vi "CreateSeriesMapFile.vi"() -> ()   [LabVIEW 2024]
panel:
  in  "Filter":string
  out "Current State":string
  in  "save key set":bool
  in  "match selected":bool
  in  "Marvel Series":i32(listbox)
  in  "Marvel Filter":i32(listbox)
  in  "CLZ Series":i32(listbox)
  in  "CLZ Filter":i32(listbox)
  in  "Exit":bool
  # "#TODO: Add Hunters fuzzy toolkit"
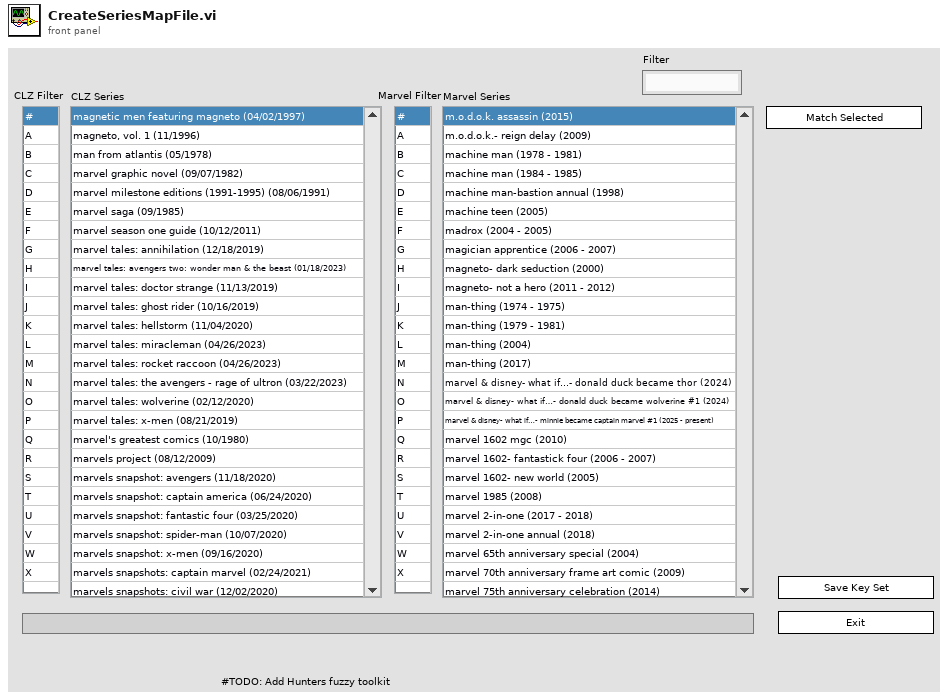
[diagram p1: front panel]
types:
  T1 = enum32{"Invalid", "Standard", "Closed", "Hidden", "Minimized", "Maximized"}
  T2 = enum32{"invalid app kind", "Development System", "Run Time System", "Student Edition", "Embedded LabVIEW", "Evaluation", "Custom"}
  T3 = cluster{"Core":cluster{"Current VI Reference":refnum<vi>, "Close Panel on Exit?":bool}, "marvel series map":map{i32, string}, "clz series map":map{i32, cluster{"series title":string, "pub date":string}}, "filtered clz map":map{string, i32}, "filtered marvel map":map{string, i32}, "key set":set{cluster{"clz.key":i32, "marvel.key":i32}}}
  T4 = map{i32, cluster{"series title":string, "pub date":string}}
  T5 = cluster{"Current VI Reference":refnum<vi>, "Close Panel on Exit?":bool}
  T6 = cluster{"key_pairs":cluster{"clz.key":i32, "marvel.key":i32}[]}
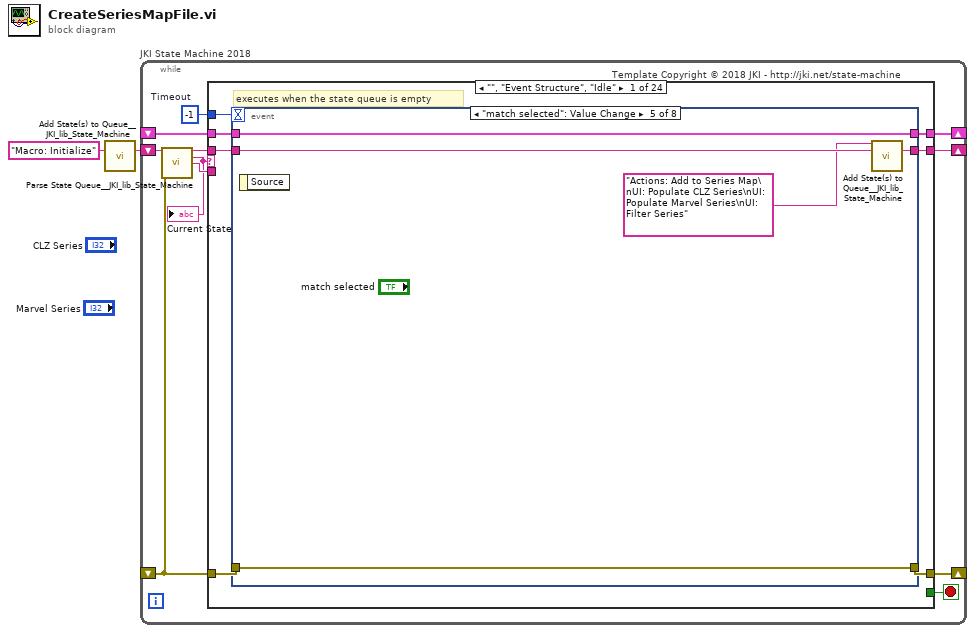
[diagram p0: block diagram]
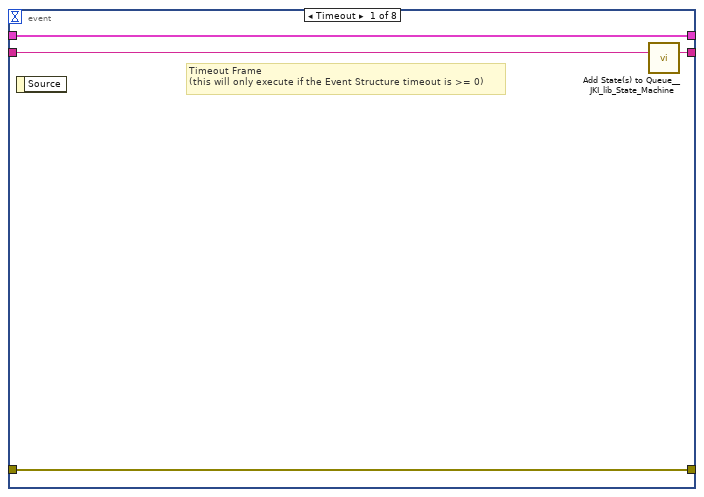
[diagram p2: hidden frame]
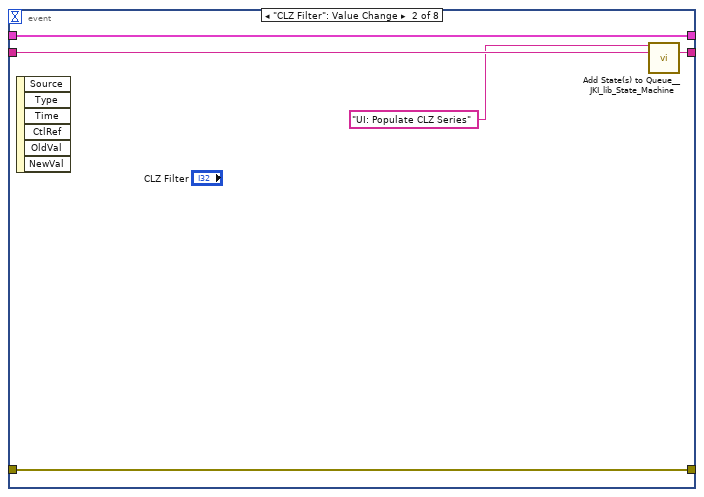
[diagram p3: hidden frame]
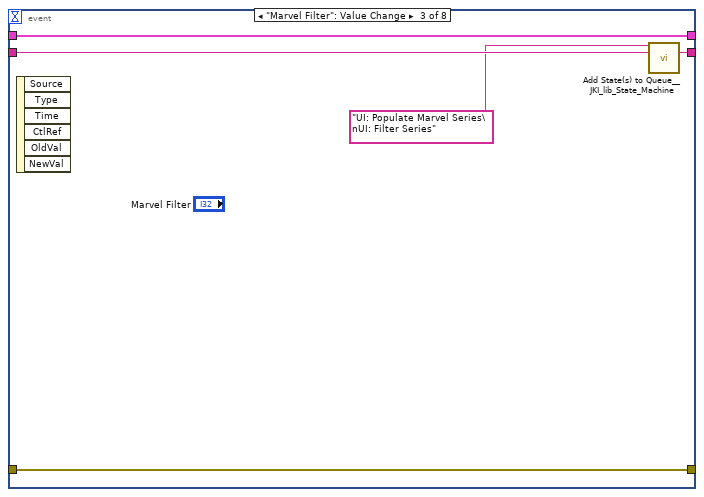
[diagram p4: hidden frame]
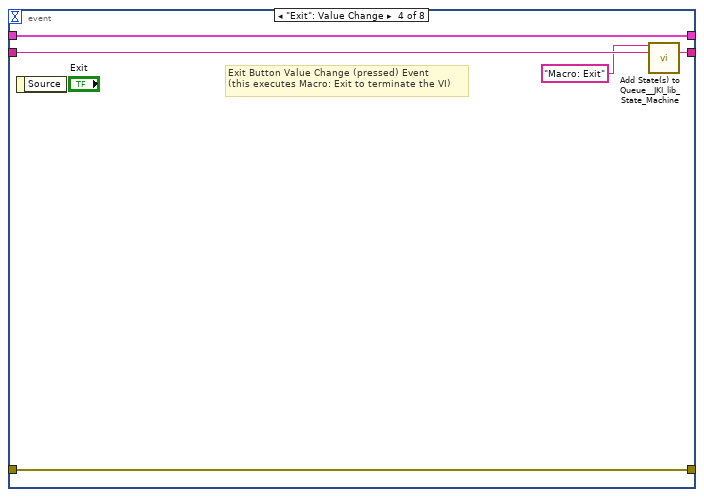
[diagram p5: hidden frame]
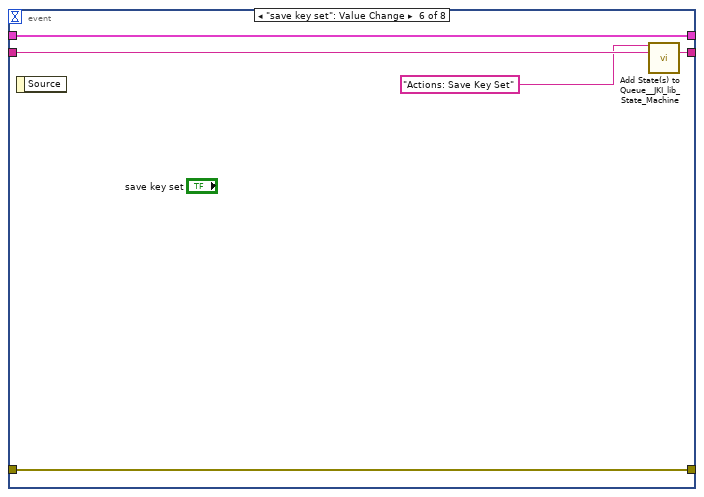
[diagram p6: hidden frame]
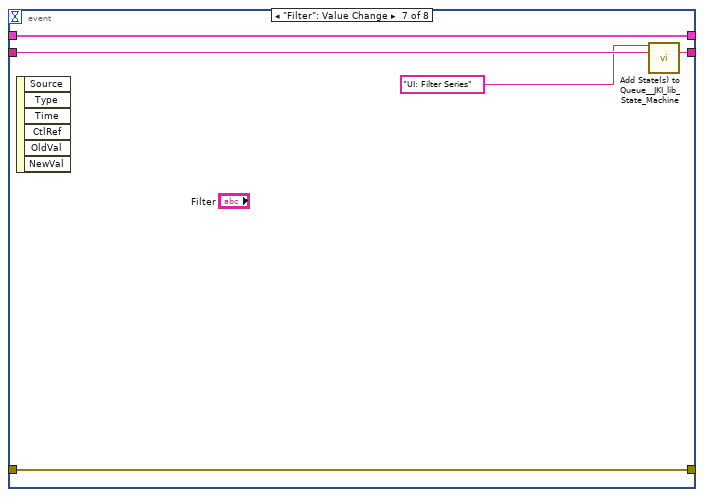
[diagram p7: hidden frame]
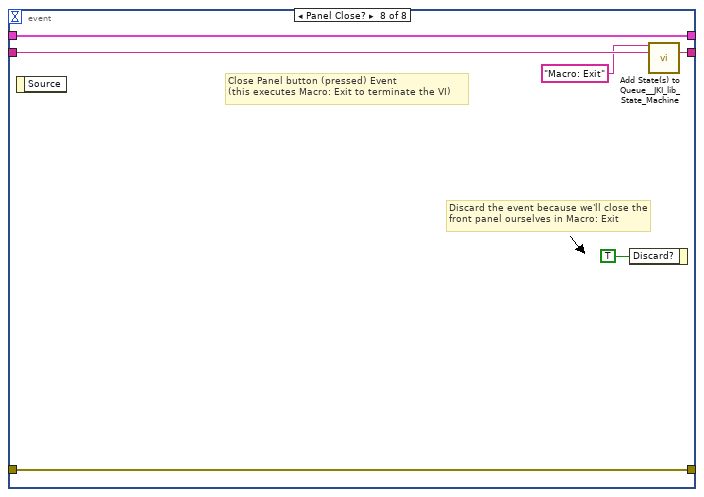
[diagram p8: hidden frame]
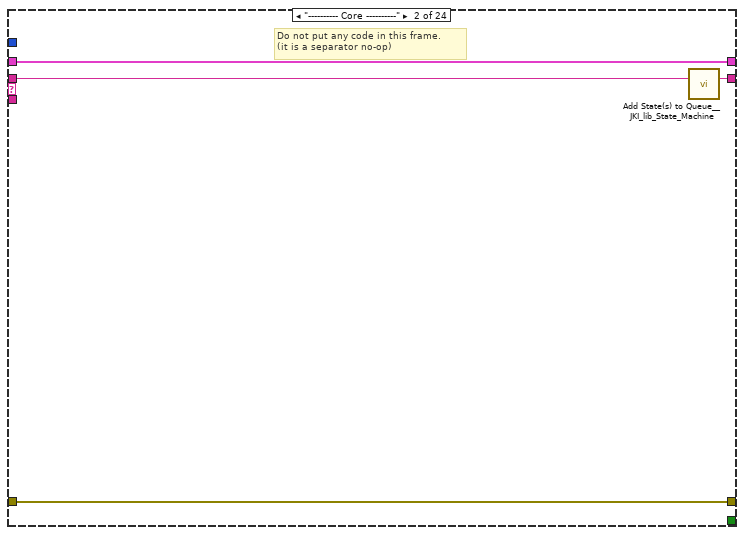
[diagram p9: hidden frame]
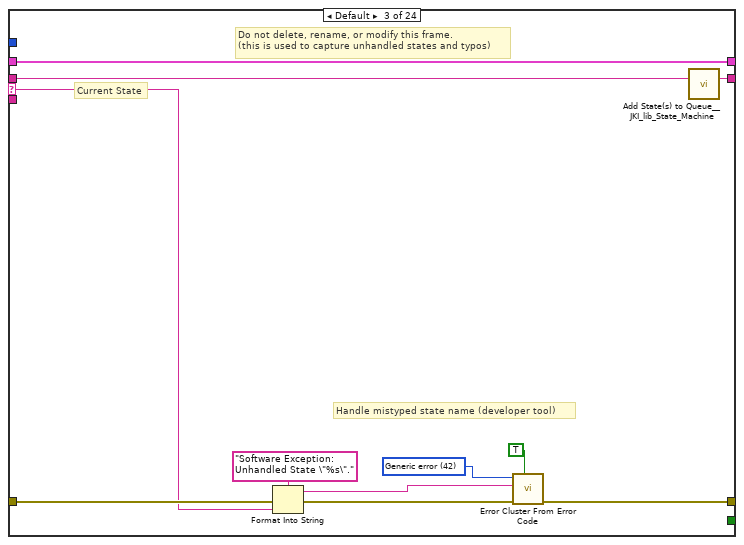
[diagram p10: hidden frame]
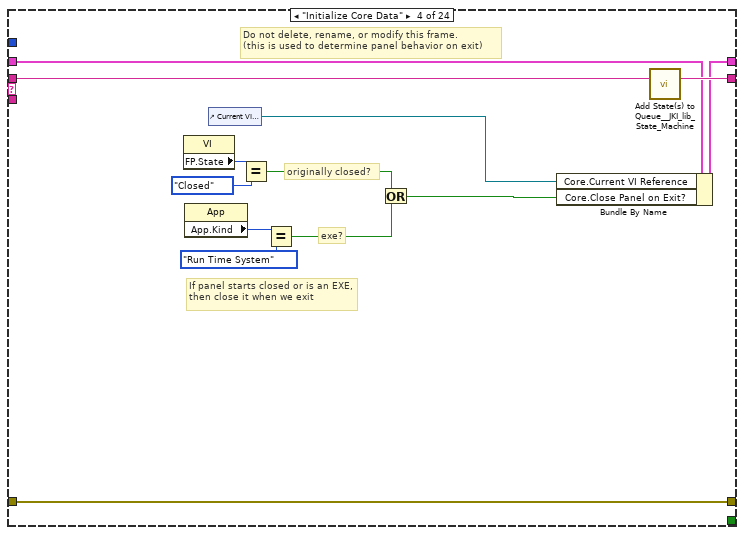
[diagram p11: hidden frame]
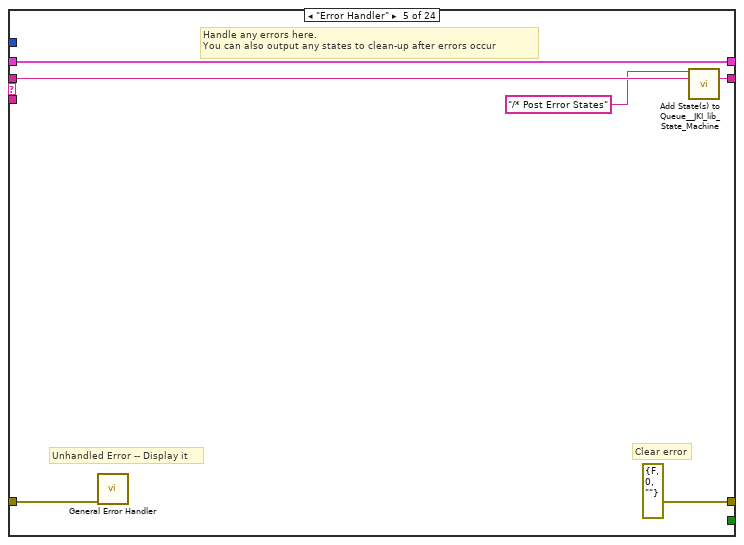
[diagram p12: hidden frame]
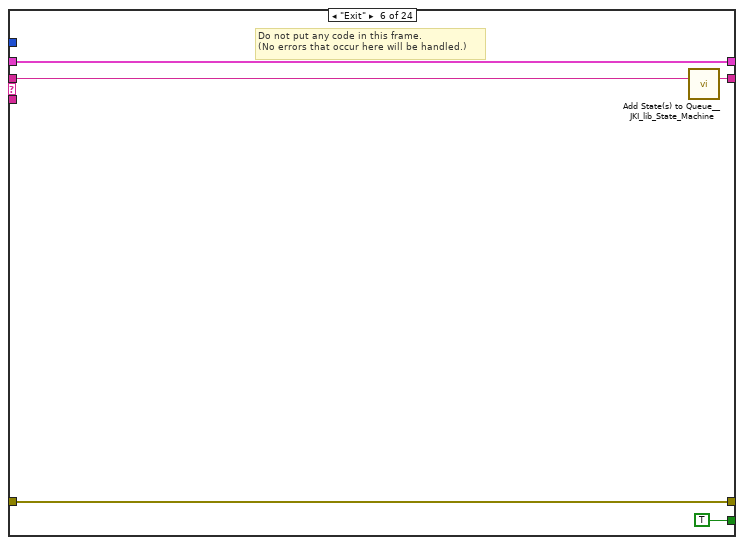
[diagram p13: hidden frame]
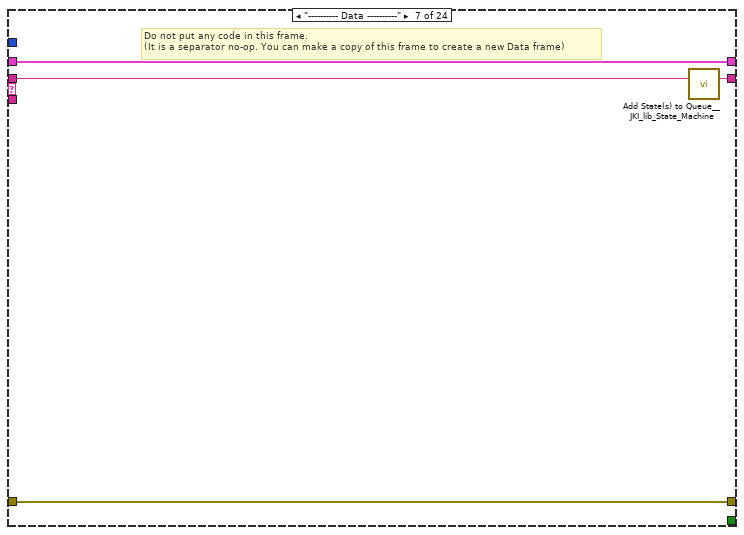
[diagram p14: hidden frame]
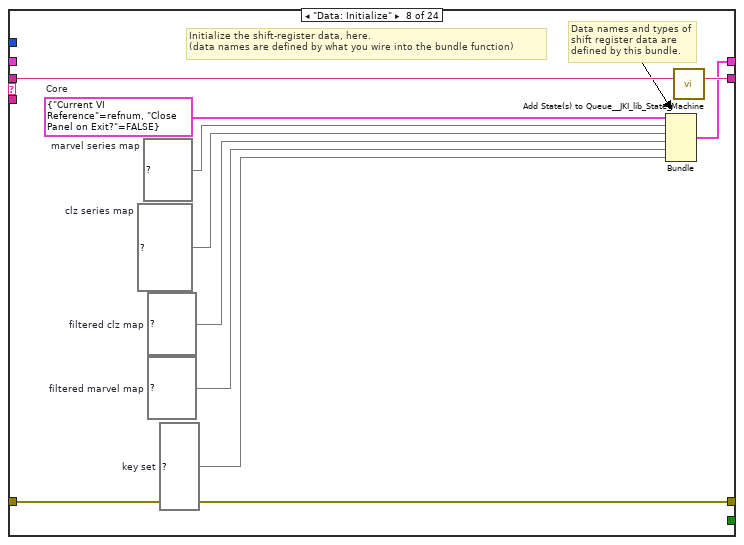
[diagram p15: hidden frame]
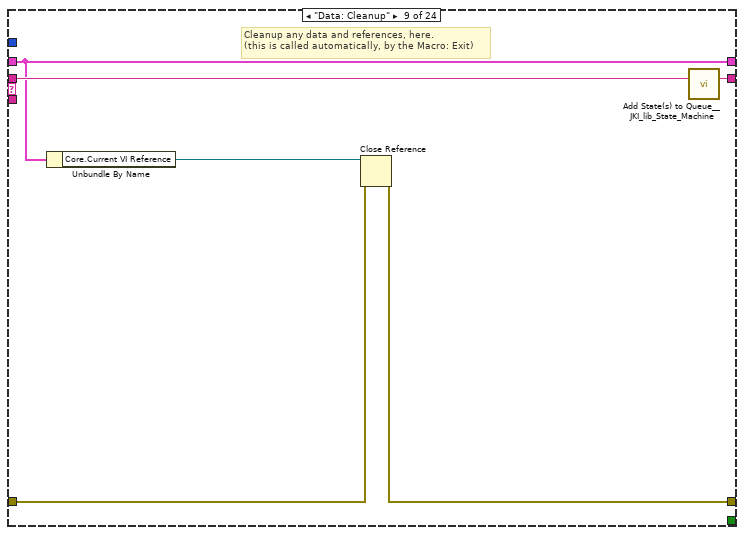
[diagram p16: hidden frame]
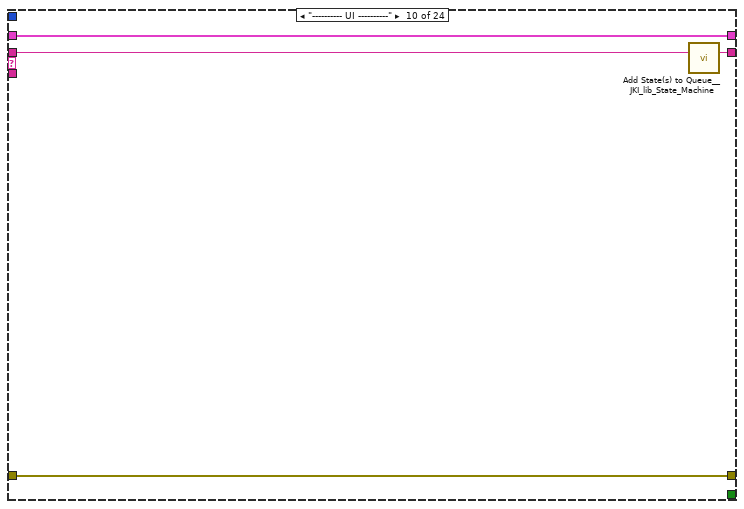
[diagram p17: hidden frame]
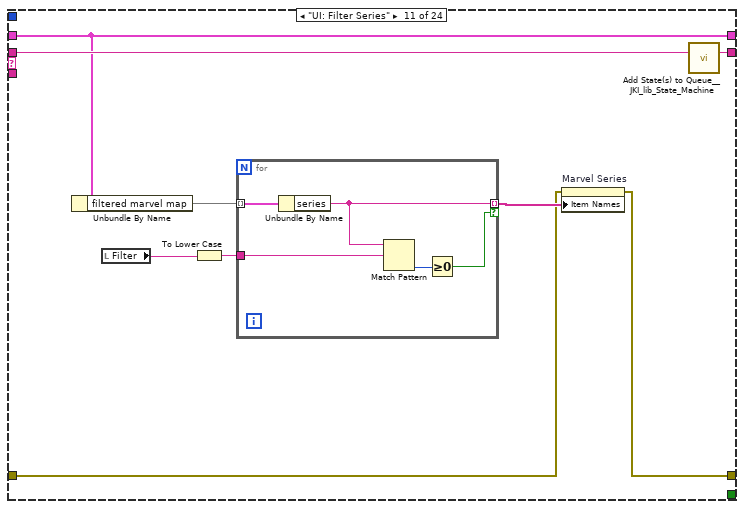
[diagram p18: hidden frame]
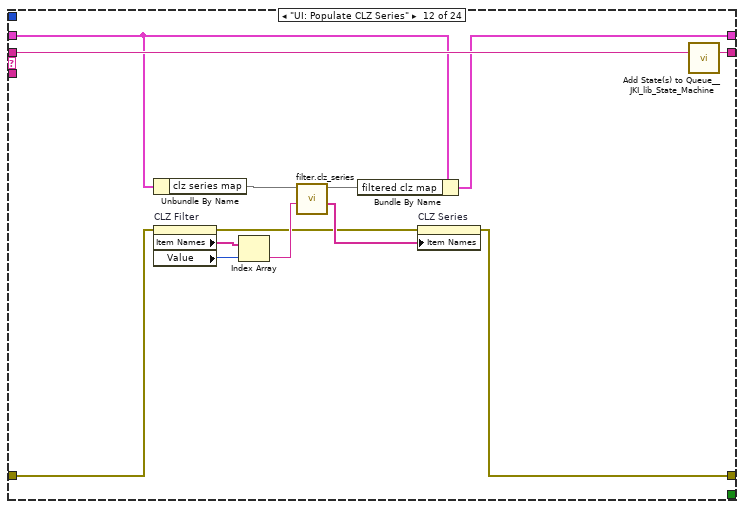
[diagram p19: hidden frame]
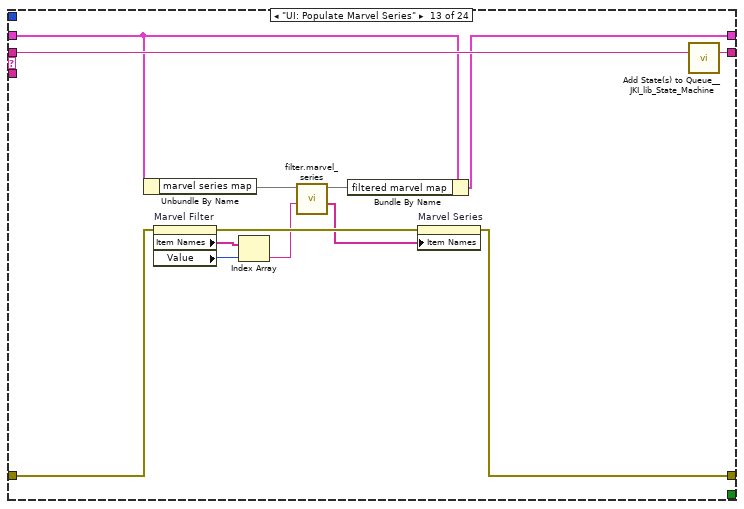
[diagram p20: hidden frame]
diagram:
  n1 = call <vilib>:"Add State(s) to Queue__JKI_lib_State_Machine.vi"("State(s) in (\"\")"="Macro: Initialize") -> ("States Out"=w2:string)  [unwired: 14 in]
  n2 = while "JKI State Machine 2018" {
    shift-right: [w7] -> _
    shift-left: _ -> [w6]
    shift-right: [w10] -> _
    shift-left: _ -> [w4]
    shift-right: [w9] -> _
    shift-left: w2 -> [w11]
    stop <- w8 stop-if-true
    w5 = -1  # Timeout
    # "Template Copyright © 2018 JKI - http://jki.net/state-machine"
    n3 = call <vilib>:"Parse State Queue__JKI_lib_State_Machine.vi"("State Queue"=w11, "Error In (no error)"=w4) -> ("Remaining States"=w13:string, "Current State"=w3:string, "Arguments"=w12:string)  [unwired: 11 in]
    "Current State" <- w3
    n4 = case shown="\"\", \"Event Structure\", \"Idle\"" w3 {
      selector: w3 -> [_ _ w65 _ _ _ _ _ _ _ _ _ _ _ _ _ _ _ _ _ _ _ _ _]
      tunnel: w13 -> [w20 w64 w69 w88 w94 w99 w103 w113 w119 w123 w132 w150 w163 w173 w179 w190 w259 w264 w274 w278 w289 w300 w316 w336]
      tunnel: w12 -> [_ _ _ _ _ _ _ _ _ _ _ _ _ _ w174 w184 _ _ _ _ _ _ _ _]
      tunnel: w6 -> [w18 w61 w67 w81 w91 w97 w100 _ w114 w120 w128 w140 w156 w171 w177 w186 w256 w261 w271 w275 w287 w292 w314 w324]
      tunnel: [w17 w62 w71 w85 errorcluster {"status"=FALSE, "code"=0, "source"=""} ("error out") w96 w101 w110 w115 w121 w124 w142 w158 w164 w175 w187 w257 w262 w272 w276 w284 w296 w301 w334] -> w10
      tunnel: w4 -> [w16 w62 w70 w85 w90 w96 w101 w110 w116 w121 w125 w141 w157 w167 w176 w188 w257 w262 w272 w276 w283 w298 w302 w334]
      tunnel: [w19 w63 w68 w87 w93 w98 w102 w112 w118 w122 w131 w149 w162 w172 w178 w189 w258 w263 w273 w277 w288 w299 w315 w335] -> w9
      tunnel: [_ _ _ _ _ TRUE _ _ _ _ _ _ _ _ _ _ _ _ _ _ _ _ _ _] -> w8
      tunnel: [w15 w61 w67 w86 w91 w97 w100 w111 w114 w120 w128 w139 w155 w171 w177 w186 w256 w261 w271 w275 w287 w295 w313 w323] -> w7
      tunnel: w5 -> [w14 _ _ _ _ _ _ _ _ _ _ _ _ _ _ _ _ _ _ _ _ _ _ _]
      frame "", "Event Structure", "Idle" {
        # "executes when the state queue is empty"
        n5 = event shown="[4] \"match selected\": Value Change" {
          selector: _ -> [_ _ _ _ _ _ _ _]
          dyn-events: _ -> [_ _ _ _ _ _ _ _]
          timeout: w14 -> [_ _ _ _ _ _ _ _]
          tunnel: w20 -> [w24 w29 w34 w39 w44 w49 w54 w60]
          tunnel: [w23 w28 w33 w38 w43 w48 w53 w59] -> w19
          tunnel: w18 -> [w21 w26 w31 w36 w41 w46 w51 w57]
          tunnel: [w22 w27 w32 w37 w42 w47 w52 w58] -> w17
          tunnel: w16 -> [w22 w27 w32 w37 w42 w47 w52 w58]
          tunnel: [w21 w26 w31 w36 w41 w46 w51 w57] -> w15
          event Timeout {
            # "Timeout Frame\n(this will only execute if the Event Structure timeout is >= 0)"
            n6 = event-data() -> ()  [unwired: 1 in, 1 out]
            n7 = call <vilib>:"Add State(s) to Queue__JKI_lib_State_Machine.vi"("State(s) in (\"\")"=w24) -> ("States Out"=w23:string)  [unwired: 14 in]
          }
          event "CLZ Filter": Value Change {
            n8 = event-data() -> ()  [unwired: 1 in, 6 out]
            n9 = call <vilib>:"Add State(s) to Queue__JKI_lib_State_Machine.vi"("State(s) in Front (\"\")"="UI: Populate CLZ Series", "State(s) in (\"\")"=w29) -> ("States Out"=w28:string)  [unwired: 13 in]
          }
          event "Marvel Filter": Value Change {
            n10 = event-data() -> ()  [unwired: 1 in, 6 out]
            n11 = call <vilib>:"Add State(s) to Queue__JKI_lib_State_Machine.vi"("State(s) in Front (\"\")"="UI: Populate Marvel Series\nUI: Filter Series", "State(s) in (\"\")"=w34) -> ("States Out"=w33:string)  [unwired: 13 in]
          }
          event "Exit": Value Change {
            # "Exit Button Value Change (pressed) Event\n(this executes Macro: Exit to terminate the VI)"
            n12 = event-data() -> ()  [unwired: 1 in, 1 out]
            n13 = call <vilib>:"Add State(s) to Queue__JKI_lib_State_Machine.vi"("State(s) in Front (\"\")"="Macro: Exit", "State(s) in (\"\")"=w39) -> ("States Out"=w38:string)  [unwired: 13 in]
          }
          event "match selected": Value Change {
            n14 = event-data() -> ()  [unwired: 1 in, 1 out]
            n15 = call <vilib>:"Add State(s) to Queue__JKI_lib_State_Machine.vi"("State(s) in Front (\"\")"="Actions: Add to Series Map\nUI: Populate CLZ Series\nUI: Populate Marvel Series\nUI: Filter Series", "State(s) in (\"\")"=w44) -> ("States Out"=w43:string)  [unwired: 13 in]
          }
          event "save key set": Value Change {
            n16 = event-data() -> ()  [unwired: 1 in, 1 out]
            n17 = call <vilib>:"Add State(s) to Queue__JKI_lib_State_Machine.vi"("State(s) in Front (\"\")"="Actions: Save Key Set", "State(s) in (\"\")"=w49) -> ("States Out"=w48:string)  [unwired: 13 in]
          }
          event "Filter": Value Change {
            n18 = event-data() -> ()  [unwired: 1 in, 6 out]
            n19 = call <vilib>:"Add State(s) to Queue__JKI_lib_State_Machine.vi"("State(s) in Front (\"\")"="UI: Filter Series", "State(s) in (\"\")"=w54) -> ("States Out"=w53:string)  [unwired: 13 in]
          }
          event Panel Close? {
            # "Discard the event because we'll close the front panel ourselves in Macro: Exit"
            # "Close Panel button (pressed) Event\n(this executes Macro: Exit to terminate the VI)"
            n20 = event-data() -> ()  [unwired: 1 in, 1 out]
            n21 = event-data("Discard?"=TRUE) -> ()  [unwired: 1 in, 1 out]
            n22 = call <vilib>:"Add State(s) to Queue__JKI_lib_State_Machine.vi"("State(s) in Front (\"\")"="Macro: Exit", "State(s) in (\"\")"=w60) -> ("States Out"=w59:string)  [unwired: 13 in]
          }
        }
      }
      frame "---------- Core ----------" {
        # "Do not put any code in this frame.\n(it is a separator no-op)"
        n23 = call <vilib>:"Add State(s) to Queue__JKI_lib_State_Machine.vi"("State(s) in (\"\")"=w64) -> ("States Out"=w63:string)  [unwired: 14 in]
      }
      frame Default {
        w74 = 42 items=["No error", "Argument error", "Memory is full", "Out of zone", "End of file", "File already open", "Generic file I/O error", "File not found", "File permission error", "Disk is full", "Duplicate path", "Too many files open", "System feature not enabled", "Resource file not found", "Cannot add resource", "Resource not found", "Image not found", "Image memory error", "Pen does not exist", "Config type invalid", "Config token not found", "Config parse error", "Config memory error", "Bad external code format", "Bad external code offset", "External code not present", "Null window", "Destroy window error", "Null menu", "Print aborted", "Bad print record", "Print driver error", "Windows error during printing", "Memory error during printing", "Print dialog error", "Generic print error", "Invalid device refnum", "Device not found", "Device parameter error", "Device unit error", "Cannot open device", "Device call aborted", "Generic error", "Cancelled by user", "Object ID too low", "Object ID too high", "Object not in heap", "Unknown heap", "Unknown object (invalid DefProc)", "Unknown object (DefProc not in table)", "Message out of range", "Invalid (null) method", "Unknown message", "Manager call not supported", "Bad address", "Network operation in progress", "Network operation timed out", "Connection is busy", "Network attribute not supported", "Network error", "Address in use", "System out of memory", "Connection aborted", "Connection refused", "Not connected", "Already connected", "Connection closed", "Initialization error (interapplication manager)", "Bad occurrence", "Wait on unbound occurrence handler", "Occurrence queue overflow", "Datalog type conflict", "Unused", "Unrecognized type (interapplication manager)", "Memory corrupt", "Failed to make temporary DLL", "Old CIN version", "Drag socket not found", "Failed to load drop-object", "Failed to register OLE object", "Failed to release OLE object", "Format specifier type mismatch", "Unknown format specifier", "Too few format specifiers", "Too many format specifiers", "Scan failed", "Newer CIN version", "Error converting to variant", "Runtime menu error", "Password tampered", "Variant attribute not found", "Incompatible variant data type", "Event data is not available", "Event Store is not present", "Occurrence is not found", "Event Queue is not created", "Event info is not available", "Refnum passed is NULL", "Error retrieving Class GUID", "Error retrieving CoClass GUID", "Error retrieving TypeLib GUID.", "Bad built application magic bytes.", "Specific driver is different from the specific driver associated with the Logical Name.", "There is no session opened to the class driver.", "Max Error", "MAX - Error with config objects", "MAX - Error loading configuration", "MAX - Group not supported"]
        # "Current State"
        # "Do not delete, rename, or modify this frame.\n(this is used to capture unhandled states and typos)"
        # "Handle mistyped state name (developer tool)"
        n24 = Format Into String(format string="Software Exception: Unhandled State \"%s\"." ("message"), error in=w70, w65) -> (resulting string=w73:string, error out=w72:errorcluster)  [unwired: 1 in]
        n25 = call <vilib>:"Error Cluster From Error Code.vi"("show call chain? (False)"=TRUE, "error in (no error)"=w72, "error message (\"\")"=w73, "error code (0)"=w74) -> ("error out"=w71:errorcluster)  [unwired: 5 in]
        n26 = call <vilib>:"Add State(s) to Queue__JKI_lib_State_Machine.vi"("State(s) in (\"\")"=w69) -> ("States Out"=w68:string)  [unwired: 14 in]
      }
      frame "Initialize Core Data" {
        # "Do not delete, rename, or modify this frame.\n(this is used to determine panel behavior on exit)"
        # "originally closed?"
        # "exe?"
        # "If panel starts closed or is an EXE, then close it when we exit"
        n27 = property class="VI"() -> ("FP.State"=w78:T1)  [unwired: 2 in, 2 out]
        n28 = property class="App"() -> ("App.Kind"=w84:T2)  [unwired: 2 in, 2 out]
        n29 = control-ref of="Current VI Reference"() -> (w79:refnum<vi>)
        n30 = Equal?(x=w78, y=T1."Closed" ("Front Panel Window:State")) -> (x = y?=w76:bool)
        n31 = Equal?(x=w84, y=T2."Run Time System" ("Application:Kind")) -> (x = y?=w82:bool)
        n32 = Or(x=w76, y=w82) -> (x .or. y?=w80:bool)
        n33 = Bundle By Name(cluster=w81, "Core.Current VI Reference"=w79, "Core.Close Panel on Exit?"=w80) -> (w86:T3)
        n34 = call <vilib>:"Add State(s) to Queue__JKI_lib_State_Machine.vi"("State(s) in (\"\")"=w88) -> ("States Out"=w87:string)  [unwired: 14 in]
      }
      frame "Error Handler" {
        # "Unhandled Error -- Display it"
        # "Handle any errors here.\nYou can also output any states to clean-up after errors occur"
        # "Clear error"
        n35 = call <vilib>:"General Error Handler.vi"("error in (no error)"=w90) -> ()  [unwired: 10 in, 5 out]
        n36 = call <vilib>:"Add State(s) to Queue__JKI_lib_State_Machine.vi"("State(s) in Front (\"\")"="/* Post Error States", "State(s) in (\"\")"=w94) -> ("States Out"=w93:string)  [unwired: 13 in]
      }
      frame "Exit" {
        # "Do not put any code in this frame.\n(No errors that occur here will be handled.)"
        n37 = call <vilib>:"Add State(s) to Queue__JKI_lib_State_Machine.vi"("State(s) in (\"\")"=w99) -> ("States Out"=w98:string)  [unwired: 14 in]
      }
      frame "---------- Data ----------" {
        # "Do not put any code in this frame.\n(It is a separator no-op. You can make a copy of this frame to create a new Data frame)"
        n38 = call <vilib>:"Add State(s) to Queue__JKI_lib_State_Machine.vi"("State(s) in (\"\")"=w103) -> ("States Out"=w102:string)  [unwired: 14 in]
      }
      frame "Data: Initialize" {
        w104 = set{cluster{"clz.key":i32, "marvel.key":i32}} {}  # key set
        w105 = map{string, i32} {}  # filtered marvel map
        w106 = map{string, i32} {}  # filtered clz map
        w107 = T4 {}  # clz series map
        w108 = map{i32, string} {}  # marvel series map
        w109 = T5 {"Current VI Reference"=refnum, "Close Panel on Exit?"=FALSE}  # Core
        # "Data names and types of shift register data are defined by this bundle."
        # "Initialize the shift-register data, here.\n(data names are defined by what you wire into the bundle function)"
        n39 = Bundle("Core"=w109, "marvel series map"=w108, "clz series map"=w107, "filtered clz map"=w106, "filtered marvel map"=w105, "key set"=w104) -> (w111:T3)  [unwired: 1 in]
        n40 = call <vilib>:"Add State(s) to Queue__JKI_lib_State_Machine.vi"("State(s) in (\"\")"=w113) -> ("States Out"=w112:string)  [unwired: 14 in]
      }
      frame "Data: Cleanup" {
        # "Cleanup any data and references, here.\n(this is called automatically, by the Macro: Exit)"
        n41 = Unbundle By Name(w114) -> ("Core.Current VI Reference"=w117:refnum<vi>)
        n42 = Close Reference(reference=w117, error in (no error)=w116) -> (error out=w115:errorcluster)
        n43 = call <vilib>:"Add State(s) to Queue__JKI_lib_State_Machine.vi"("State(s) in (\"\")"=w119) -> ("States Out"=w118:string)  [unwired: 14 in]
      }
      frame "---------- UI ----------" {
        n44 = call <vilib>:"Add State(s) to Queue__JKI_lib_State_Machine.vi"("State(s) in (\"\")"=w123) -> ("States Out"=w122:string)  [unwired: 14 in]
      }
      frame "UI: Filter Series" {
        n45 = Unbundle By Name(w128) -> ("filtered marvel map"=w127:map{string, i32})
        n46 = local read "Filter"() -> (w129:string)
        n47 = To Lower Case(string=w129) -> (all lower case string=w130:string)
        n48 = for {
          tunnel: w127 -> [w137] mode=indexing
          tunnel: w130 -> [w136]
          tunnel: [w135] -> w126 mode=indexing if=w133
          n49 = Unbundle By Name(w137) -> ("series"=w135:string)
          n50 = Match Pattern(string=w135, regular expression=w136) -> (offset past match=w134:i32)  [unwired: 1 in, 3 out]
          n51 = Greater Or Equal To 0?(x=w134) -> (x >= 0?=w133:bool)
        }
        n52 = property on="Marvel Series" class="LstBox (strict)"(error in=w125, "Item Names"=w126) -> (error out=w124:errorcluster)  [unwired: 1 in, 1 out]
        n53 = call <vilib>:"Add State(s) to Queue__JKI_lib_State_Machine.vi"("State(s) in (\"\")"=w132) -> ("States Out"=w131:string)  [unwired: 14 in]
      }
      frame "UI: Populate CLZ Series" {
        n54 = Unbundle By Name(w140) -> ("clz series map"=w146:T4)
        n55 = property on="CLZ Filter" class="LstBox (strict)"(error in=w141) -> (error out=w143:errorcluster, "Item Names"=w148:string[], "Value"=w147:i32)  [unwired: 1 in, 1 out]
        n56 = Index Array(array=w148, index=w147) -> (element=w145:string)
        n57 = call "filter.clz_series.vi"("filter char"=w145, "clz series map"=w146) -> ("series array"=w144:string[], "series map out"=w138:map{string, i32})  [unwired: 8 in]
        n58 = Bundle By Name(cluster=w140, "filtered clz map"=w138) -> (w139:T3)
        n59 = property on="CLZ Series" class="LstBox (strict)"(error in=w143, "Item Names"=w144) -> (error out=w142:errorcluster)  [unwired: 1 in, 1 out]
        n60 = call <vilib>:"Add State(s) to Queue__JKI_lib_State_Machine.vi"("State(s) in (\"\")"=w150) -> ("States Out"=w149:string)  [unwired: 14 in]
      }
      frame "UI: Populate Marvel Series" {
        n61 = Unbundle By Name(w156) -> ("marvel series map"=w154:map{i32, string})
        n62 = property on="Marvel Filter" class="LstBox (strict)"(error in=w157) -> (error out=w159:errorcluster, "Item Names"=w161:string[], "Value"=w160:i32)  [unwired: 1 in, 1 out]
        n63 = Index Array(array=w161, index=w160) -> (element=w152:string)
        n64 = call "filter.marvel_series.vi"("filter char"=w152, "marvel series map"=w154) -> ("series array"=w151:string[], "series map out"=w153:map{string, i32})  [unwired: 8 in]
        n65 = Bundle By Name(cluster=w156, "filtered marvel map"=w153) -> (w155:T3)
        n66 = property on="Marvel Series" class="LstBox (strict)"(error in=w159, "Item Names"=w151) -> (error out=w158:errorcluster)  [unwired: 1 in, 1 out]
        n67 = call <vilib>:"Add State(s) to Queue__JKI_lib_State_Machine.vi"("State(s) in (\"\")"=w163) -> ("States Out"=w162:string)  [unwired: 14 in]
      }
      frame "UI: Initialize" {
        # "Initialize the User Interface, here.\n(this is called automatically, by the Macro: Init)"
        n68 = call "GenerateAlphabetArray.vi"() -> ("Array"=w169:string[])
        n69 = Build Array (concatenate)("#", w169) -> (w168:string[])
        n70 = property on="Marvel Filter" class="LstBox (strict)"(error in=w167, "Item Names"=w168) -> (error out=w165:errorcluster)  [unwired: 1 in, 1 out]
        n71 = property on="Marvel Filter" class="LstBox (strict)"(error in=w167, "Item Names"=w168) -> (error out=w166:errorcluster)  [unwired: 1 in, 1 out]
        n72 = Merge Errors(w165, w166) -> (w164:errorcluster)
        n73 = call <vilib>:"Add State(s) to Queue__JKI_lib_State_Machine.vi"("State(s) in (\"\")"=w173) -> ("States Out"=w172:string)  [unwired: 14 in]
      }
      frame "UI: Cursor Set" {
        # "Argument"
        # "Set and Unset Cursor Busy.\n(Usage: \"UI: Cursor Set >> Busy|Idle\")"
        n74 = case shown="\"Idle\", Default" w174 {
          tunnel: w176 -> [w181 w183]
          tunnel: [w180 w182] -> w175
          frame "Idle", Default {
            n75 = call <vilib>:"Unset Busy.vi"("error in (no error)"=w181) -> ("error out"=w180:errorcluster)  [unwired: 10 in]
          }
          frame "Busy" {
            n76 = call <vilib>:"Set Busy.vi"("error in (no error)"=w183) -> ("error out"=w182:errorcluster)  [unwired: 9 in, 1 out]
          }
        }
        n77 = call <vilib>:"Add State(s) to Queue__JKI_lib_State_Machine.vi"("State(s) in (\"\")"=w179) -> ("States Out"=w178:string)  [unwired: 14 in]
      }
      frame "UI: Front Panel State" {
        # "Argument"
        # "Set Front Panel Open or Closed\n(Usage: \"UI: Front Panel State >> Open|Close\")"
        n78 = Unbundle By Name(w186) -> ("Core.Current VI Reference"=w185:refnum<vi>)
        n79 = case shown="\"Minimize\", \"Minimized\"" w184 {
          tunnel: w188 -> [w196 w211 w222 w235 w248]
          tunnel: [w198 w212 w224 w237 w250] -> w187
          tunnel: w185 -> [w197 w209 w223 w236 w249]
          frame "Open", "Standard", Default {
            w191 = T1."Standard" ("State")
            n80 = property class="VI"(reference=w197, error in=w196) -> (reference out=w194:refnum<vi>, error out=w195:errorcluster, "FP.State"=w193:T1)
            n81 = Not Equal?(x=w193, y=w191) -> (x != y?=w192:bool)
            n82 = case shown="True" w192 {
              tunnel: [w202 w204] -> w198
              tunnel: w195 -> [w201 w204]
              tunnel: w194 -> [w200 _]
              tunnel: w191 -> [w199 _]
              frame True {
                n83 = invoke class="VI" method="FP.Open"(reference=w200, error in=w201, "Activate"=TRUE, "State"=w199) -> (error out=w202:errorcluster)  [unwired: 1 in, 4 out]
              }
              frame False {
              }
            }
          }
          frame "Close", "Closed" {
            n84 = property class="VI"(reference=w209, error in=w211) -> (reference out=w208:refnum<vi>, error out=w210:errorcluster, "FP.State"=w206:T1)
            n85 = Not Equal?(x=w206, y=T1."Closed" ("Front Panel Window:State")) -> (x != y?=w205:bool)
            n86 = case shown="True" w205 {
              tunnel: [w213 w216] -> w212
              tunnel: w210 -> [w213 w215]
              tunnel: w208 -> [_ w214]
              frame False {
              }
              frame True {
                n87 = invoke class="VI" method="FP.Close"(reference=w214, error in=w215) -> (error out=w216:errorcluster)  [unwired: 1 in, 2 out]
              }
            }
          }
          frame "Hidden", "Hide" {
            w217 = T1."Hidden" ("State")
            n88 = property class="VI"(reference=w223, error in=w222) -> (reference out=w220:refnum<vi>, error out=w221:errorcluster, "FP.State"=w219:T1)
            n89 = Not Equal?(x=w219, y=w217) -> (x != y?=w218:bool)
            n90 = case shown="True" w218 {
              tunnel: [w228 w229] -> w224
              tunnel: w221 -> [w227 w229]
              tunnel: w220 -> [w226 _]
              tunnel: w217 -> [w225 _]
              frame True {
                n91 = invoke class="VI" method="FP.Open"(reference=w226, error in=w227, "State"=w225) -> (error out=w228:errorcluster)  [unwired: 2 in, 4 out]
              }
              frame False {
              }
            }
          }
          frame "Minimize", "Minimized" {
            w230 = T1."Minimized" ("State")
            n92 = property class="VI"(reference=w236, error in=w235) -> (reference out=w233:refnum<vi>, error out=w234:errorcluster, "FP.State"=w232:T1)
            n93 = Not Equal?(x=w232, y=w230) -> (x != y?=w231:bool)
            n94 = case shown="True" w231 {
              tunnel: [w241 w242] -> w237
              tunnel: w234 -> [w240 w242]
              tunnel: w233 -> [w239 _]
              tunnel: w230 -> [w238 _]
              frame True {
                n95 = invoke class="VI" method="FP.Open"(reference=w239, error in=w240, "State"=w238) -> (error out=w241:errorcluster)  [unwired: 2 in, 4 out]
              }
              frame False {
              }
            }
          }
          frame "Maximize", "Maximized" {
            w243 = T1."Maximized" ("State")
            n96 = property class="VI"(reference=w249, error in=w248) -> (reference out=w246:refnum<vi>, error out=w247:errorcluster, "FP.State"=w245:T1)
            n97 = Not Equal?(x=w245, y=w243) -> (x != y?=w244:bool)
            n98 = case shown="True" w244 {
              tunnel: [w254 w255] -> w250
              tunnel: w247 -> [w253 w255]
              tunnel: w246 -> [w252 _]
              tunnel: w243 -> [w251 _]
              frame True {
                n99 = invoke class="VI" method="FP.Open"(reference=w252, error in=w253, "State"=w251) -> (error out=w254:errorcluster)  [unwired: 2 in, 4 out]
              }
              frame False {
              }
            }
          }
        }
        n100 = call <vilib>:"Add State(s) to Queue__JKI_lib_State_Machine.vi"("State(s) in (\"\")"=w190) -> ("States Out"=w189:string)  [unwired: 14 in]
      }
      frame "---------- Macro ----------" {
        # "Do not put any code in this frame.\n(It is a separator no-op. You can make a copy of this frame to create a new Macro frame)"
        n101 = call <vilib>:"Add State(s) to Queue__JKI_lib_State_Machine.vi"("State(s) in (\"\")"=w259) -> ("States Out"=w258:string)  [unwired: 14 in]
      }
      frame "Macro: Initialize" {
        # "Initialization Macro\n(This is called once, when the VI starts)"
        n102 = call <vilib>:"Add State(s) to Queue__JKI_lib_State_Machine.vi"("State(s) in Front (\"\")"="UI: Cursor Set >> Busy\nData: Initialize\nInitialize Core Data\nUI: Initialize\nActions: Load Key Set\nActions: Load Series Maps\nUI: Populate CLZ Series\nUI: Populate Marvel Series\nUI: Front Panel State >> Open\nUI: Cursor Set >> Idle", "State(s) in (\"\")"=w264) -> ("States Out"=w263:string)  [unwired: 13 in]
      }
      frame "Macro: Exit" {
        # "Exit Macro\n(This is called once, when the VI exits)"
        n103 = Unbundle By Name(w271) -> ("Core.Close Panel on Exit?"=w270:bool)
        n104 = Select(t="UI: Front Panel State >> Close", s=w270, f="") -> (s? t:f=w267:string)
        n105 = call <vilib>:"Add State(s) to Queue__JKI_lib_State_Machine.vi"("State(s) in (\"\")"=w267, "State(s) at Back (\"\")"="Data: Cleanup\nExit") -> ("States Out"=w265:string)  [unwired: 13 in]
        n106 = call <vilib>:"Add State(s) to Queue__JKI_lib_State_Machine.vi"("State(s) in Front (\"\")"=w265, "State(s) in (\"\")"=w274) -> ("States Out"=w273:string)  [unwired: 13 in]
      }
      frame "---------- Actions ----------" {
        n107 = call <vilib>:"Add State(s) to Queue__JKI_lib_State_Machine.vi"("State(s) in (\"\")"=w278) -> ("States Out"=w277:string)  [unwired: 14 in]
      }
      frame "Actions: Save Key Set" {
        w281 = T6 {"key_pairs"=[]}  # key_pair_array
        n108 = Unbundle By Name(w287) -> ("key set"=w282:set{cluster{"clz.key":i32, "marvel.key":i32}})
        n109 = for {
          tunnel: w282 -> [w290] mode=indexing
          tunnel: [w290] -> w280 mode=indexing
        }
        n110 = Bundle By Name(cluster=w281, "key_pairs"=w280) -> (w279:T6)
        n111 = call <vilib>:"Easy Write XML File__JKI EasyXML.vi"("error in (no error)"=w283, "Overwrite File? (false)"=TRUE, "LabVIEW Data"=w279, "XML File Path"=path "d:/data/series.set.xml") -> ("error out"=w284:errorcluster)  [unwired: 6 in, 1 out]
        n112 = call <vilib>:"Add State(s) to Queue__JKI_lib_State_Machine.vi"("State(s) in (\"\")"=w289) -> ("States Out"=w288:string)  [unwired: 14 in]
      }
      frame "Actions: Load Series Maps" {
        n113 = Unbundle By Name(w292) -> ("key set"=w291:set{cluster{"clz.key":i32, "marvel.key":i32}})
        n114 = call "GenerateMarvelSeriesMap.vi"("key set"=w291, "error in (no error)"=w298) -> ("error out"=w297:errorcluster, "map"=w294:map{i32, string})  [unwired: 8 in]
        n115 = call "GenerateCLZSeriesMap.vi"("key set"=w291, "error in (no error)"=w297) -> ("error out"=w296:errorcluster, "map"=w293:T4)  [unwired: 8 in]
        n116 = Bundle By Name(cluster=w292, "marvel series map"=w294, "clz series map"=w293) -> (w295:T3)
        n117 = call <vilib>:"Add State(s) to Queue__JKI_lib_State_Machine.vi"("State(s) in (\"\")"=w300) -> ("States Out"=w299:string)  [unwired: 14 in]
      }
      frame "Actions: Load Key Set" {
        w306 = T6 {"key_pairs"=[]}  # key_pair_array
        w312 = set{cluster{"clz.key":i32, "marvel.key":i32}} {}  # key set
        n118 = Read from Text File(file (use dialog)=path "D:/data/series.set.xml" ("XML File Path"), error in=w302) -> (text=w310:string, error out=w309:errorcluster)  [unwired: 2 in, 2 out]
        n119 = call <vilib>:"Easy Parse XML__JKI EasyXML.vi"("error in (no error)"=w309, "LabVIEW Data (Type)"=w306, "XML String"=w310) -> ("error out"=w308:errorcluster, "LabVIEW Data"=w307:variant)  [unwired: 7 in]
        n120 = Variant To Data(error in=w308, type=w306, Variant=w307) -> (data=w305:T6, error out=w301:errorcluster)
        n121 = Unbundle By Name(w305) -> ("key_pairs"=w304:cluster{"clz.key":i32, "marvel.key":i32}[])
        n122 = for {
          shift-right: [w318] -> w303
          shift-left: w312 -> [w319]
          tunnel: w304 -> [w317] mode=indexing
          n123 = Insert Into Set(10:w317, 11:w319) -> (3:w318:set{cluster{"clz.key":i32, "marvel.key":i32}})  [unwired: 1 out]
        }
        n124 = Bundle By Name(cluster=w314, "key set"=w303) -> (w313:T3)
        n125 = call <vilib>:"Add State(s) to Queue__JKI_lib_State_Machine.vi"("State(s) in (\"\")"=w316) -> ("States Out"=w315:string)  [unwired: 14 in]
      }
      frame "Actions: Add to Series Map" {
        n126 = Unbundle By Name(w324) -> ("filtered clz map"=w329:map{string, i32}, "filtered marvel map"=w328:map{string, i32})
        n127 = property on="CLZ Series" class="LstBox (strict)"() -> ("Item Names"=w333:string[], "Value"=w332:i32)  [unwired: 2 in, 2 out]
        n128 = property on="Marvel Series" class="LstBox (strict)"() -> ("Item Names"=w330:string[], "Value"=w331:i32)  [unwired: 2 in, 2 out]
        n129 = Index Array(array=w333, index=w332) -> (element=w326:string)
        n130 = Index Array(array=w330, index=w331) -> (element=w327:string)
        n131 = Look In Map(map=w329, key=w326) -> (value=w320:i32)  [unwired: 1 in, 1 out]
        n132 = Look In Map(map=w328, key=w327) -> (value=w321:i32)  [unwired: 1 in, 1 out]
        n133 = Bundle By Name(cluster=cluster{"clz.key":i32, "marvel.key":i32} {"clz.key"=0, "marvel.key"=0}, "clz.key"=w320, "marvel.key"=w321) -> (w322:cluster{"clz.key":i32, "marvel.key":i32})
        n134 = in-place {
          in-place-border: w322 -> [w343]
          in-place-border: w321 -> [w340]
          in-place-border: w320 -> [w337]
          n135 = in-place-cluster #1(w324) -> ("marvel series map"=w342:map{i32, string}, "clz series map"=w339:T4, "key set"=w345:set{cluster{"clz.key":i32, "marvel.key":i32}})
          n136 = Remove From Map(10:w340, 11:w342) -> (3:w341:map{i32, string})  [unwired: 2 out]
          n137 = Insert Into Set(10:w343, 11:w345) -> (3:w344:set{cluster{"clz.key":i32, "marvel.key":i32}})  [unwired: 1 out]
          n138 = Remove From Map(10:w337, 11:w339) -> (3:w338:T4)  [unwired: 2 out]
          n139 = in-place-cluster #1("marvel series map"=w341, "clz series map"=w338, "key set"=w344) -> (w323:T3)
        }
        n140 = call <vilib>:"Add State(s) to Queue__JKI_lib_State_Machine.vi"("State(s) in (\"\")"=w336) -> ("States Out"=w335:string)  [unwired: 14 in]
      }
    }
  }
